vi "Dock UI.vi"(8 "error in (no error)":errorcluster, 11 "picoG in":refnum<class "picoG.lvclass">) -> (0 "error out":errorcluster, 3 "picoG out":refnum<class "picoG.lvclass">)   [LabVIEW 2020, in "PicoG-App.lvlib" / "picoG.lvclass"]
uses:
  picoG.lvclass
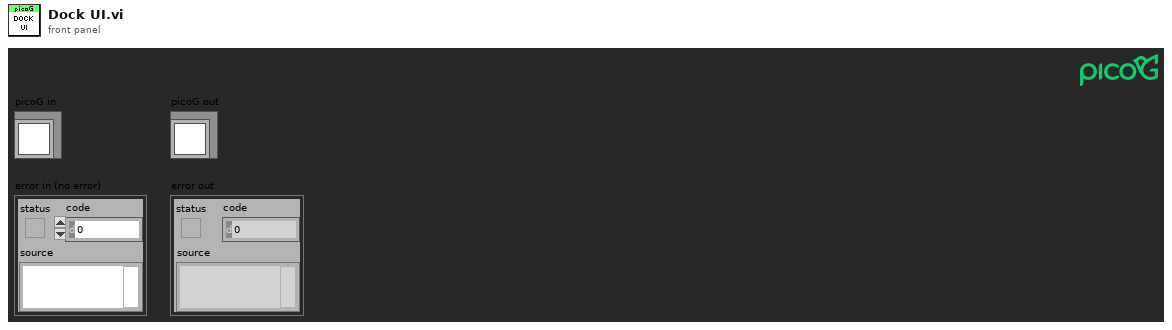
[diagram p1: front panel]
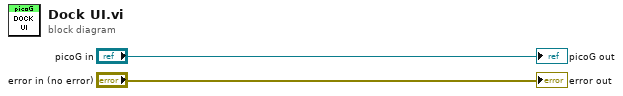
[diagram p0: block diagram]
diagram:
  "error out" <- "error in (no error)"
  "picoG out" <- "picoG in"
